vi "Switch Check.vi"(8 "error in (no error)":errorcluster, 11 "Switch Schedule":T1) -> (0 "error out":errorcluster)   [LabVIEW 2014]
doc: "Checks all entries in the Switch Schedule for any actions that must occur."
uses:
  Controls/Switch Schedule.ctl
  Controls/Switch Program.ctl
  Controls/Action Enum.ctl
  Controls/Switch Day.ctl
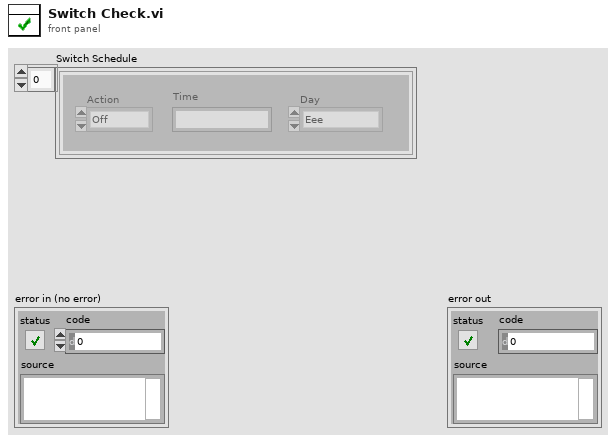
[diagram p1: front panel]
types:
  T1 = typedef "Switch Schedule.ctl" = T2[]
  T2 = typedef "Switch Program.ctl" = cluster{"Action":T3, "Time":string, "Day":T4}
  T3 = typedef "Action Enum.ctl" = enum16{"Off", "On"}
  T4 = typedef "Switch Day.ctl" = enum16{"Eee", "Sun", "Mon", "Tue", "Wed", "Thu", "Fri", "Sat"}
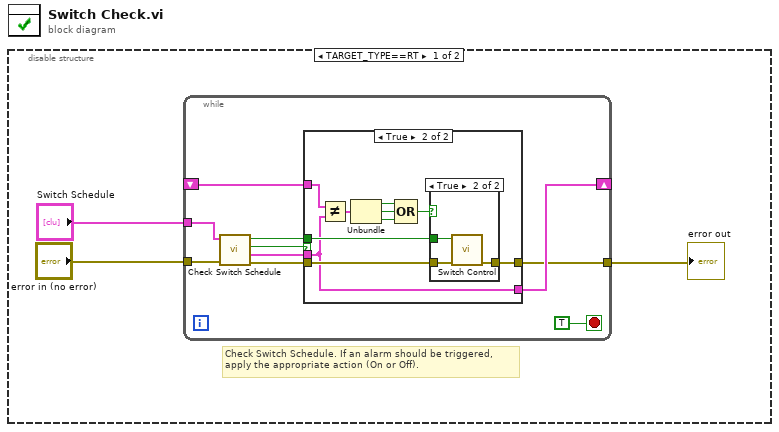
[diagram p0: block diagram]
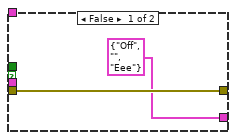
[diagram p2: hidden frame]
diagram:
  n1 = disable-structure shown="TARGET_TYPE==RT" {
    frame condition #0 (active) {
      # "Check Switch Schedule. If an alarm should be triggered,\napply the appropriate action (On or Off)."
      n2 = while {
        tunnel: "Switch Schedule" -> [w8]
        tunnel: [w7] -> w2
        tunnel: "error in (no error)" -> [w5]
        shift-right: [w12] -> _
        shift-left: _ -> [w13]
        stop <- TRUE stop-if-true
        n3 = call "Check Switch Schedule.vi"("error in (no error)"=w5, "Switch Schedule"=w8) -> ("error out"=w6:errorcluster, "Switch Program"=w11:T2, "Trigger?"=w10:bool, "On/Off"=w9:bool)  [unwired: 6 in]
        n4 = case shown="True" w10 {
          tunnel: w6 -> [w15 w25]
          tunnel: [w15 w24] -> w7
          tunnel: w9 -> [_ w23]
          tunnel: w11 -> [_ w17]
          tunnel: [T2 {"Action"=enum."Off", "Time"="", "Day"=enum."Eee"} ("Switch Program") w17] -> w12
          tunnel: w13 -> [_ w16]
          frame False {
          }
          frame True {
            n5 = Not Equal?(x=w16, y=w17) -> (x != y?=w22:cluster{"Action":bool, "Time":bool, "Day":bool})
            n6 = Unbundle(w22) -> ("Action"=w20:bool, "Time"=w21:bool, "Day"=w19:bool)
            n7 = Compound Arithmetic op=OR(w20, w21, w19) -> (w18:bool)
            n8 = case shown="True" w18 {
              tunnel: w25 -> [w26 w29]
              tunnel: [w26 w28] -> w24
              tunnel: w23 -> [_ w27]
              frame False {
              }
              frame True {
                n9 = call "Switch Control.vi"("error in (no error)"=w29, "On/Off"=w27) -> ("error out"=w28:errorcluster)  [unwired: 9 in]
              }
            }
          }
        }
      }
      "error out" <- w2
    }
    frame condition #1 {
    }
  }
